vi "Chart[Template].METHOD_TEMPLATE.vi"(8 "error in (no error)":errorcluster, 10 "Data In":string, 11 "DisplayWaveforms":refnum<class "DisplayWaveforms.lvclass">) -> (0 "error out":errorcluster, 2 "Data Out":string, 3 "DisplayWaveforms out":refnum<class "DisplayWaveforms.lvclass">)   [LabVIEW 2018, in "DisplayWaveform.lvlib" / "DisplayWaveforms.lvclass"]
doc: "---------------------------------------------------------------\nJKI State Machine Objects™\nhttp://jki.net/state-machine-objects/\nCopyright (C) 2005-2015, JKI <info@jki.net>\nALL RIGHTS RESERVEDJKI State Machine Objects (SMO) 1.0.0.5\nJKI - JKI\nCopyright (c) 2016, JKI"
uses:
  DisplayWaveforms.lvclass
panel:
  # "For instructions on how to use the JKI State Machine Objects, examples and video tutorials, visit:\nhttp://jki.net/state-machine-objects/\n\nJKI State Machine Objects™\nhttp://jki.net/state-machine-objects/\nCopyright (C) 2005-2015, JKI <info@jki.net>\nALL RIGHTS RESERVED"
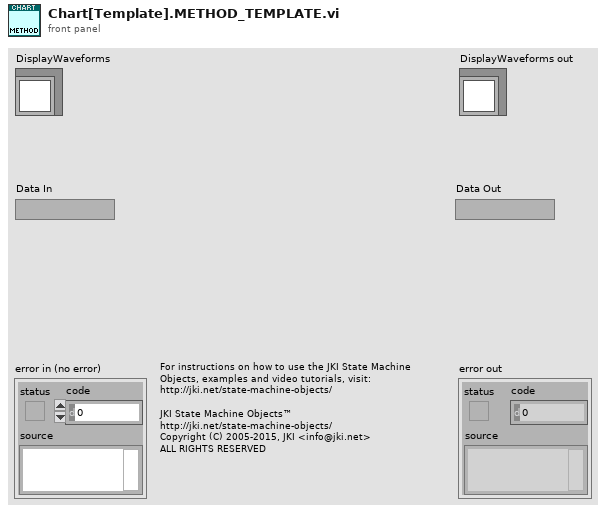
[diagram p1: front panel]
types:
  T1 = typedef "DisplayWaveform.lvlib/DisplayWaveforms.lvclass/PrivateData--Ref.ctl" = refnum<data-value>
  T2 = typedef "DisplayWaveform.lvlib/DisplayWaveforms.lvclass/PrivateData--Cluster.ctl" = cluster{"Public Events":T3, "Protected Events":T4, "Data":string, "Dependencies":T5}
  T3 = typedef "DisplayWaveform.lvlib/DisplayWaveforms.lvclass/PublicEvents--Cluster.ctl" = cluster{"Chart Cleared":refnum<user-event>, "Chart Exported":refnum<user-event>, "ChartParams Set":refnum<user-event>}
  T4 = typedef "DisplayWaveform.lvlib/DisplayWaveforms.lvclass/ProtectedEvents--Cluster.ctl" = cluster{"Clear Chart":refnum<user-event>, "Pause Chart":refnum<user-event>, "Update Chart":refnum<user-event>, "Export Chart":refnum<user-event>, "Set ChartParams":refnum<user-event>}
  T5 = typedef "DisplayWaveform.lvlib/DisplayWaveforms.lvclass/Dependencies--Cluster.ctl" = cluster{"New Value":refnum<user-event>}
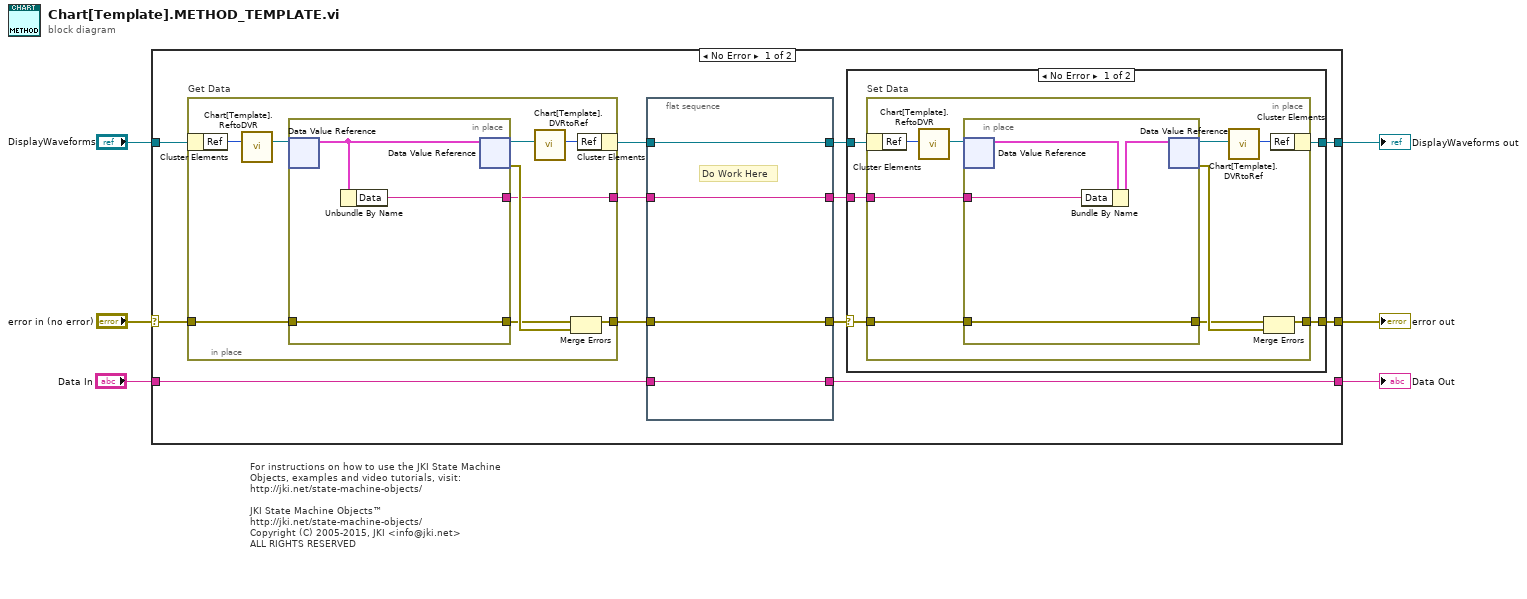
[diagram p0: block diagram]
diagram:
  # "For instructions on how to use the JKI State Machine Objects, examples and video tutorials, visit:\nhttp://jki.net/state-machine-objects/\n\nJKI State Machine Objects™\nhttp://jki.net/state-machine-objects/\nCopyright (C) 2005-2015, JKI <info@jki.net>\nALL RIGHTS RESERVED"
  n1 = case shown="No Error" "error in (no error)" {
    selector: "error in (no error)" -> [w17 w56]
    tunnel: "DisplayWaveforms" -> [w18 w57]
    tunnel: [w13 w56] -> w5
    tunnel: [w12 w57] -> w4
    tunnel: [w11 w55] -> w2
    tunnel: "Data In" -> [w10 w55]
    frame No Error {
      n2 = in-place "Get Data" {
        in-place-border: w17 -> [w51]
        in-place-border: [w48] -> w15
        in-place-border: [w47] -> w8
        n3 = in-place-cluster #1(w18) -> ("Ref"=w46:u32)
        n4 = call "Chart[Template].ReftoDVR.vi"("Ref"=w46) -> ("Ref"=w45:T1)  [unwired: 10 in]
        n5 = in-place {
          in-place-border: w51 -> [w53]
          in-place-border: [w53] -> w49
          in-place-border: [w52] -> w47
          n6 = in-place-dvr #2(w45) -> (w54:T2)  [unwired: 1 out]
          n7 = Unbundle By Name(w54) -> ("Data"=w52:string)
          n8 = in-place-dvr #2(w54) -> (w44:T1, w50:errorcluster)
        }
        n9 = call "Chart[Template].DVRtoRef.vi"("Ref"=w44) -> ("Ref"=w43:u32)  [unwired: 10 in]
        n10 = Merge Errors(w49, w50) -> (w48:errorcluster)
        n11 = in-place-cluster #1("Ref"=w43) -> (w16:refnum<class "DisplayWaveforms.lvclass">)
      }
      n12 = flat-sequence {
        tunnel: w16 -> [w42]
        tunnel: [w42] -> w14
        tunnel: w15 -> [w41]
        tunnel: [w41] -> w7
        tunnel: [w40] -> w11
        tunnel: w10 -> [w40]
        tunnel: [w39] -> w9
        tunnel: w8 -> [w39]
        frame #0 {
          # "Do Work Here"
        }
      }
      n13 = case shown="No Error" w7 {
        selector: w7 -> [w19 w37]
        tunnel: w14 -> [w23 w38]
        tunnel: [w22 w37] -> w13
        tunnel: [w21 w38] -> w12
        tunnel: w9 -> [w20 _]
        frame No Error {
          n14 = in-place "Set Data" {
            in-place-border: w19 -> [w32]
            in-place-border: [w29] -> w22
            in-place-border: w20 -> [w28]
            n15 = in-place-cluster #3(w23) -> ("Ref"=w27:u32)
            n16 = call "Chart[Template].ReftoDVR.vi"("Ref"=w27) -> ("Ref"=w26:T1)  [unwired: 10 in]
            n17 = in-place {
              in-place-border: w32 -> [w35]
              in-place-border: [w35] -> w30
              in-place-border: w28 -> [w33]
              n18 = in-place-dvr #4(w26) -> (w36:T2)  [unwired: 1 out]
              n19 = Bundle By Name(cluster=w36, "Data"=w33) -> (w34:T2)
              n20 = in-place-dvr #4(w34) -> (w25:T1, w31:errorcluster)
            }
            n21 = call "Chart[Template].DVRtoRef.vi"("Ref"=w25) -> ("Ref"=w24:u32)  [unwired: 10 in]
            n22 = Merge Errors(w30, w31) -> (w29:errorcluster)
            n23 = in-place-cluster #3("Ref"=w24) -> (w21:refnum<class "DisplayWaveforms.lvclass">)
          }
        }
        frame Error {
          # "Do not write back on error"
        }
      }
    }
    frame Error {
    }
  }
  "error out" <- w5
  "DisplayWaveforms out" <- w4
  "Data Out" <- w2
